vi "Image to String.vi"() -> ()   [LabVIEW 2015]
panel:
  out "Color Palette out":cluster{"Red":u8, "Green":u8, "Blue":u8}[](array[cluster])
  out "Image":T1(plugin-control)
  out "Data String":string
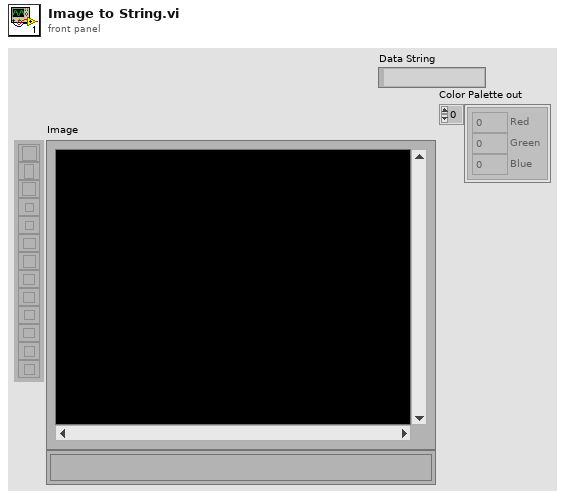
[diagram p1: front panel]
types:
  T1 = typedef "IMAQ Image.ctl" = refnum<image>
  T2 = typedef "Image Type" = u32
  T3 = cluster{"Read Raw File":i32, "File Data Type":u32, "Offset to Data":i32, "Use Min Max":enum32{"Don't use min max", "Use file values", "Use optional values"}, "Optional Min Value":sgl, "Optional Max Value":sgl, "Byte Order":enum32{"Big endian (Motorola)", "Little endian (Intel)"}}
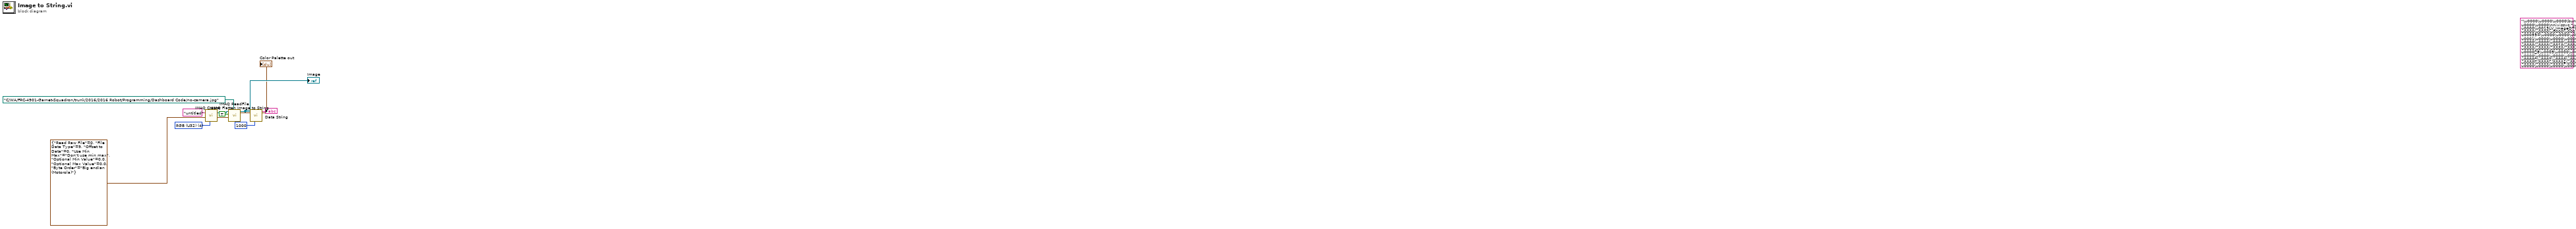
[diagram p0: block diagram]
diagram:
  w1 = T2 4 items=["Grayscale (U8)", "Grayscale (I16)", "Grayscale (SGL)", "Complex (CSG)", "RGB (U32)", "HSL (U32)", "RGB (U64)", "Grayscale (U16)"] ("Image Type")
  (unwired) "\u0000\u0000\u0000\buntitled\u0000\u0000\u0000\nnivissvc.*\u0000\u0000\u0000\u0013LV_ImageDTClassInfo\u0000\u0000\u0000\u0001\u0000\u00059=\u0000\u0000\u0010\u0000\u0001\u0000\u0000\u0000\u0000\u0000\u0000\u0000\u0000\u0000\u0000\u0000\u0000\u0000\u0010\u0000¬\u0000\u0000\u0000\u0000\u0000\u0000\u00008\u0005\u0000\u0000\u0000\u0000\u0000\u0000\u0000\u0000\u0000\u0002\u0000\u0000\u0000\u0000\u0000\u0000à\u0001\u0000\u0000\u0000\u0000\u0000\u0000\u0003\u0000\u0000\u0000\u0000\u0000\u0000\u0000\u0000\u0000\u0000\u0000\u0000\u0000\u0000\u0000\u0000\u0000\u0000\u0000\u0000\u0000\u0000\u0000\u0000\u0000\u0000\u0000À\u0002\u0000\u0000\u0000\u0000\u0000\u0000\u0000\u0000\u0000\u0000\u0010\u0003E\n\u0000\u0000\u0000\u0000,ºc\u000f\u0000\u0000\u0000\u0000\u0000\u0005<z\u0000\u0000\u0000\b<\u0000\u0000\u0000\u0000\u0000\u0000\u0000\u0000\u0000\u0000\u0001\u0000\u0000\u0000\u0001\u0000\u0000\u0000\u0000\u0000\u0000\u0000\b\u0000\u0000\u00008\u0005\u0000\u0000\u0000\u0000\u0000\u0000\u0000\u0000\u0000\u0000\u0000\u0000\u0000\t\u0000\u0000\u0000\u0000\u0000\u0000\u0000untitled\u0000\u0000\u0000\u0000\u0000\u0000\u0000\u0000\u0000\u0000\u0000\u0000\u0000\u0000\u0000\u0000\u0000\u0000\u0000\u0000\u0000\u0000\u0000\u0000\u0000\u0000\u0000\u0000\u0000\u0000\u0000\u0000\u0000\u0000\u0000\u0000\u0000\u0000\u0000\u0000\u0000\u0000\u0000\u0000\u0000\u0000\u0000\u0000\u0000\u0000\u0000\u0000\u0000\u0000\u0000\u0000\u0000\u0000\u0000\u0000\u0000\u0000\u0000\u0000\u0000\u0000\u0000\u0000\u0000\u0002\u0000\u0000\u0000\u0002\u0000\u0000\u0000\u0002\u0000\u0000\u0000\u0002\u0000\u0000\u0000\u0002\u0000\u0000\u0000\u0002\u0000\u0000\u0000\u0002\u0000\u0000\u0000\u0002\u0000\u0000\u0000\u0002\u0000\u0000\u0000\u0002\u0000\u0000\u0000\u0002\u0000\u0000\u0000\u0002\u0000\u0000\u0000\u0002\u0000\u0000\u0000\u0002\u0000\u0000\u0000\u0002\u0000\u0000\u0000\u0002\u0000\u0000\u0000\u0002\u0000\u0000\u0000\u0002\u0000\u0000\u0000\u0002\u0000\u0000\u0000\u0002\u0000\u0000\u0000\u0002\u0000\u0000\u0000\u0002\u0000\u0000\u0000\u0002\u0000\u0000\u0000\u0002\u0000\u0000\u0000\u0002\u0000\u0000\u0000\u0002\u0000\u0000\u0000\u0002\u0000\u0000\u0000\u0002\u0000\u0000\u0000\u0002\u0000\u0000\u0000\u0002\u0000\u0000\u0000\u0002\u0000\u0000\u0000\u0002\u0000\u0000\u0000\u0002\u0000\u0000\u0000\u0002\u0000\u0000\u0000\u0002\u0000\u0000\u0000\u0002\u0000\u0000\u0000\u0002\u0000\u0000\u0000\u0002\u0000\u0000\u0000\u0002\u0000\u0000\u0000\u0002\u0000\u0000\u0000\u0002\u0000\u0000\u0000\u0002\u0000\u0000\u0000\u0002\u0000\u0000\u0000\u0002\u0000\u0000\u0000\u0002\u0000\u0000\u0000\u0002\u0000\u0000\u0000\u0002\u0000\u0000\u0000\u0002\u0000\u0000\u0000\u0002\u0000\u0000\u0000\u0002\u0000\u0000\u0000\u0002\u0000\u0000\u0000\u0002\u0000\u0000\u0000\u0002\u0000\u0000\u0000\u0002\u0000\u0000\u0000\u0002\u0000\u0000\u0000\u0002\u0000\u0000\u0000\u0002\u0000\u0000\u0000\u0002\u0000\u0000\u0000\u0002\u0000\u0000\u0000\u0002\u0000\u0000\u0000\u0002\u0000\u0000\u0000\u0002\u0000\u0000\u0000\u0002\u0000\u0000\u0000\u0002\u0000\u0001\u0000\u0002\u0000\u0001\u0000\u0002\u0000\u0001\u0000\u0002\u0000\u0001\u0000\u0002\u0000\u0001\u0000\u0002\u0000\u0001\u0000\u0002\u0000\u0001\u0000\u0002\u0000\u0001\u0000\u0002\u0000\u0001\u0000\u0002\u0000\u0001\u0000\u0002\u0000..." ("Data String")
  n1 = call "IMAQ Create"("Image Name"="untitled", "Image Type"=w1) -> ("New Image"=w10:T1)  [unwired: 3 in, 1 out]
  n2 = call "IMAQ ReadFile"("File Path"=path "C:/WA/FRC-4901-Garnet-Squadron/trunk/2016/2016 Robot/Programming/Dashboard Code/no-camera.jpg", "File Options"=T3 {"Read Raw File"=0, "File Data Type"=9, "Offset to Data"=0, "Use Min Max"=enum."Don't use min max", "Optional Min Value"=0.0, "Optional Max Value"=0.0, "Byte Order"=enum."Big endian (Motorola)"}, "Load Color Palette? (No)"=TRUE, "Image"=w10) -> ("Image Out"=w4:T1, "Color Palette out"=→"Color Palette out":cluster{"Red":u8, "Green":u8, "Blue":u8}[])  [unwired: 3 in, 3 out]
  "Image" <- w4
  n3 = call "IMAQ Flatten Image to String"("Quality (750)"=1000, "Image"=w4) -> ("Data String"=→"Data String":string)  [unwired: 8 in, 1 out]
